vi "20170502127惠雨5.vi"() -> ()   [LabVIEW 2017]
uses:
  <vilib>/Analysis/NI_AALBase.lvlib
panel:
  out "波形图":dbl[](graph)
  in  "延时（秒）":dbl(slide) scale=0.01..0.1
  in  "停止":bool
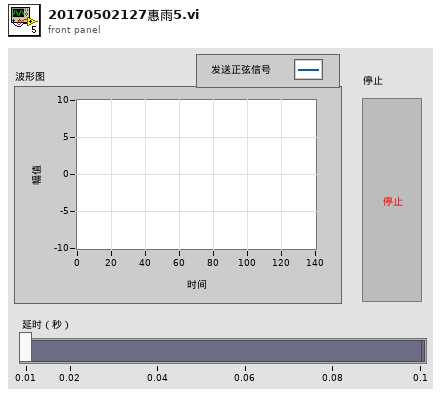
[diagram p1: front panel]
types:
  T1 = enum16{"Read", "Write", "ReadWrite", "BufferedRead", "BufferedReadWrite"}
  T2 = cluster{"Sinusoidal Pattern":dbl[], "延时（秒）":dbl, "停止":bool}
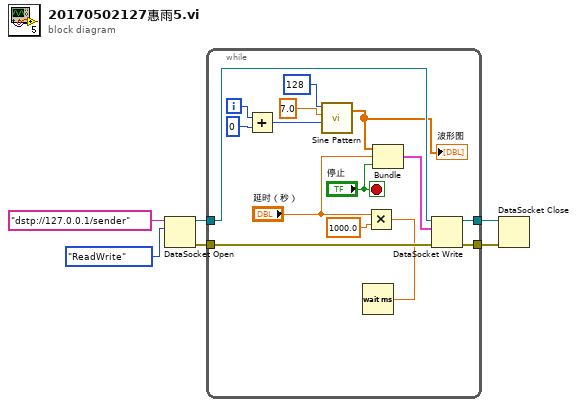
[diagram p0: block diagram]
diagram:
  n1 = DataSocket Open(10:T1."ReadWrite" ("模式"), 11:"dstp://127.0.0.1/sender" ("URL")) -> (0:w3:errorcluster, 3:w5:refnum<k13>)  [unwired: 2 in]
  n2 = while {
    tunnel: w5 -> [w21]
    tunnel: [w18] -> w4
    tunnel: w3 -> [w17]
    tunnel: [w16] -> w2
    i -> [w13]
    stop <- "停止" stop-if-true
    n3 = Add(x=w13, y=0) -> (x+y=w12:i32)
    n4 = call <vilib>:"Sine Pattern.vi"("phase(degrees)"=w12, "amplitude"=7.0, "samples"=128) -> ("Sinusoidal Pattern"=w7:dbl[])  [unwired: 1 in, 1 out]
    "波形图" <- w7
    n5 = Multiply(x="延时（秒）", y=1000.0) -> (x*y=w10:dbl)
    n6 = Wait (ms)(milliseconds to wait=w10) -> ()  [unwired: 1 out]
    n7 = Bundle("Sinusoidal Pattern"=w7, "延时（秒）"="延时（秒）", "停止"="停止") -> (w14:T2)  [unwired: 1 in]
    n8 = DataSocket Write(8:w17, 10:w14, 11:w21) -> (0:w16:errorcluster, 3:w18:refnum<k13>)  [unwired: 1 in, 1 out]
  }
  n9 = DataSocket Close(8:w2, 11:w4) -> ()  [unwired: 1 in, 2 out]
